vi "_Start.vi"(8 "error in (no error)":errorcluster, 11 "Block in":refnum<class "Block.lvclass">) -> (0 "error out":errorcluster, 3 "Block out":refnum<class "Block.lvclass">)   [LabVIEW 2020, in "Parallel Block.lvlib" / "Block.lvclass"]
uses:
  Block.lvclass
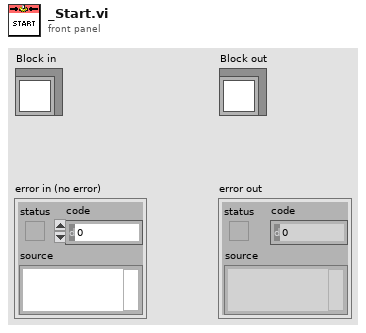
[diagram p1: front panel]
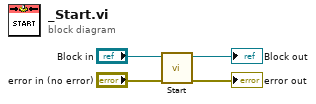
[diagram p0: block diagram]
diagram:
  n1 = call-dynamic "Start.vi"("error in (no error)"="error in (no error)", "Block in"="Block in") -> ("error out"=→"error out":errorcluster, "Block out"=→"Block out":refnum<class "Block.lvclass">)  [unwired: 8 in]
